vi "Configure.vi"(8 "error in (no error)":errorcluster, 11 "BMC in":refnum<class "BMC.lvclass">) -> (0 "error out":errorcluster, 2 "cancelled?":bool, 3 "BMC out":refnum<class "BMC.lvclass">)   [LabVIEW 2012, in "BMC.lvclass"]
doc: "The configure method configures the details for the RabbitMQ connection. \n\nIn the derived class, make a call to the parent for setting these parameters."
uses:
  BMC.lvclass
  Murmex/LabVIEW/Murmex/Murmex/Murmex.lvclass
  <vilib>/Utility/miscctls.llb/LVPointTypeDef.ctl
panel:
  in  "button::cancel":bool
  in  "button::ok":bool
  in  "button::configure Murmex":bool
  in  "Tab Control":enum32{"IDs and stati"}(tab)
  in  "pStatus":i32[](array[numeric])
  in  "Status":i32
  in  "DevId":i32
  in  "pDevideIDs":i32[](array[numeric])
  # "RabbitMQ parameters"
  # "Window position"
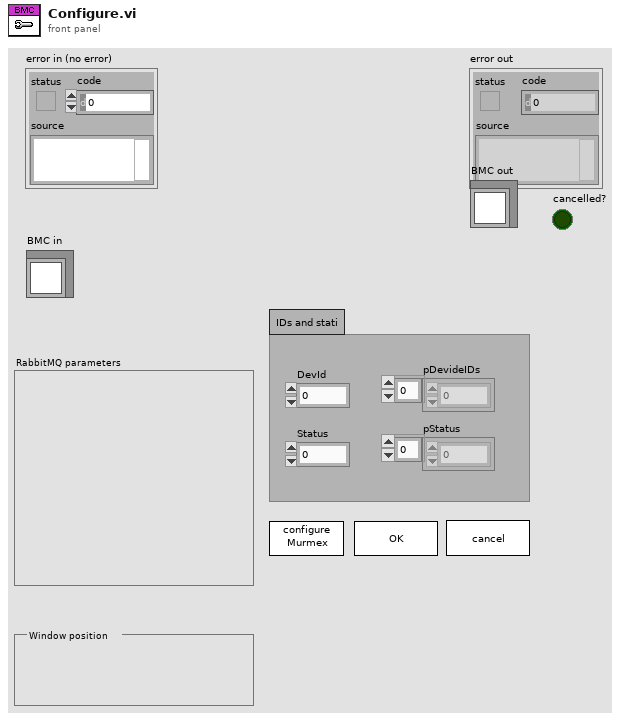
[diagram p1: front panel]
types:
  T1 = typedef "LVPointTypeDef.ctl" = cluster{"Horizontal":i16, "Vertical":i16}
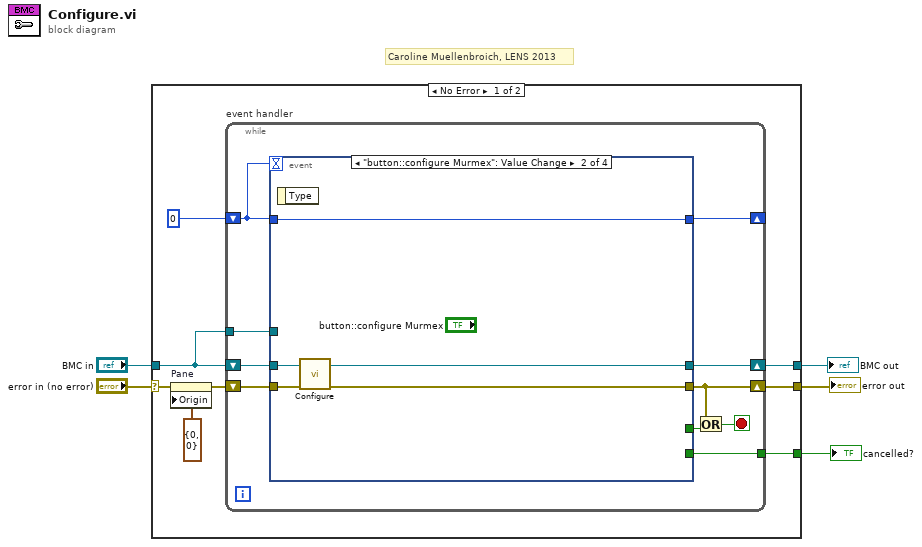
[diagram p0: block diagram]
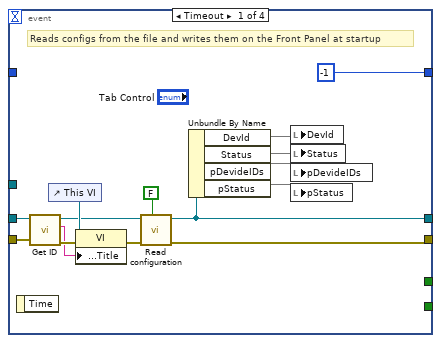
[diagram p2: hidden frame]
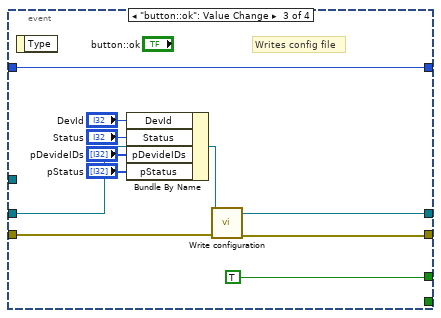
[diagram p3: hidden frame]
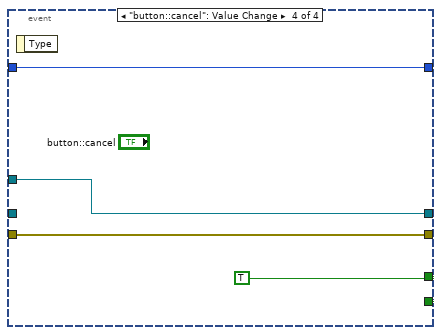
[diagram p4: hidden frame]
diagram:
  # "Caroline Muellenbroich, LENS 2013"
  n1 = case shown="No Error" "error in (no error)" {
    selector: "error in (no error)" -> [w8 w59]
    tunnel: "BMC in" -> [w13 w60]
    tunnel: [w11 w60] -> w3
    tunnel: [w10 w59] -> w2
    tunnel: [w9 _] -> w1
    frame No Error {
      n2 = property on="Pane" class="Pane"(error in=w8, "Origin"=T1 {"Horizontal"=0, "Vertical"=0}) -> (error out=w7:errorcluster)  [unwired: 1 in, 1 out]
      n3 = while "event handler" {
        shift-right: [w16] -> w10
        shift-left: w7 -> [w23]
        shift-right: [w18] -> w11
        shift-left: w13 -> [w22]
        tunnel: w13 -> [w21]
        shift-right: [w19] -> _
        shift-left: 0 -> [w20]
        tunnel: [w15] -> w9
        stop <- w17 stop-if-true
        n4 = event shown="[1] \"button::configure Murmex\": Value Change" {
          selector: _ -> [_ _ _ _]
          dyn-events: _ -> [_ _ _ _]
          timeout: w20 -> [_ _ _ _]
          tunnel: w23 -> [w38 w42 w51 w56]
          tunnel: w22 -> [w37 w40 w45 _]
          tunnel: w21 -> [_ _ _ w57]
          tunnel: w20 -> [_ w43 w54 w58]
          tunnel: [-1 w43 w54 w58] -> w19
          tunnel: [w28 w39 w52 w57] -> w18
          tunnel: [w29 w41 w53 w56] -> w16
          tunnel: [_ _ _ w55] -> w15
          tunnel: [_ _ TRUE w55] -> w14
          event Timeout {
            # "Reads configs from the file and writes them on the Front Panel at startup"
            n5 = event-data() -> ()  [unwired: 1 in, 1 out]
            n6 = call "Get ID.vi"("error in (no error)"=w38, "Murmex in"=w37) -> ("error out"=w35:errorcluster, "component id"=w30:string, "Murmex out"=w32:refnum<class "BMC.lvclass">)  [unwired: 7 in]
            n7 = control-ref of="This VI"() -> (w34:refnum<vi>)
            n8 = property class="VI"(reference=w34, error in=w35, "Front Panel.Title"=w30) -> (error out=w33:errorcluster)  [unwired: 1 out]
            n9 = call-dynamic "Read configuration.vi"("force loading?"=FALSE, "error in (no error)"=w33, "BMC in"=w32) -> ("error out"=w29:errorcluster, "BMC out"=w28:refnum<class "BMC.lvclass">)  [unwired: 7 in]
            n10 = Unbundle By Name(w28) -> ("DevId"=w27, "Status"=w26, "pDevideIDs"=w25, "pStatus"=w24)
            n11 = local write "DevId"(w27) -> ()
            n12 = local write "Status"(w26) -> ()
            n13 = local write "pDevideIDs"(w25) -> ()
            n14 = local write "pStatus"(w24) -> ()
          }
          event "button::configure Murmex": Value Change {
            n15 = event-data() -> ()  [unwired: 1 in, 1 out]
            n16 = call-parent "Configure.vi"("error in (no error)"=w42, "Murmex in"=w40) -> ("error out"=w41:errorcluster, "Murmex out"=w39:refnum<class "BMC.lvclass">)  [unwired: 7 in, 1 out]
          }
          event "button::ok": Value Change {
            # "Writes config file"
            n17 = event-data() -> ()  [unwired: 1 in, 1 out]
            n18 = Bundle By Name(cluster=w45, "DevId"="DevId", "Status"="Status", "pDevideIDs"="pDevideIDs", "pStatus"="pStatus") -> (w49:refnum<class "BMC.lvclass">)
            n19 = call-dynamic "Write configuration.vi"("error in (no error)"=w51, "BMC in"=w49) -> ("error out"=w53:errorcluster, "BMC out"=w52:refnum<class "BMC.lvclass">)  [unwired: 8 in]
          }
          event "button::cancel": Value Change {
            w55 = TRUE
            n20 = event-data() -> ()  [unwired: 1 in, 1 out]
          }
        }
        n21 = Or(x=w16, y=w14) -> (x .or. y?=w17:bool)
      }
    }
    frame Error {
    }
  }
  "error out" <- w2
  "BMC out" <- w3
  "cancelled?" <- w1
